vi "Controller Fast Command Loop.vi"(7 "Sync Objects":T1, 8 "error in (no error)":errorcluster, 11 "FOFB Configuration":T4={"FOFB Parameters"={"Network"={"FOFB Controller IP"="", "LNLS Control Network IP"="", "LNLS Control Network Power Supplies TCP Port"=0, "LNLS Control Network FOFB Configuration TCP Port"=0, "LNLS Control Network BPMs TCP Port"=0, "Data Server TCP Port"=0, "Monitoring Data TCP Port"=0, "Configuration GUI TCP Port"=0, "Storage Data TCP Port"=0, "Fast Command TCP Port"=0, "TCP Listening Timeout"=0, "Request Setpoints Rate"=0}, "Fast Acquisition"={"Acquisition Period"=0, "Data Buffer Size"=0, "Monitoring Period"=0}, "Response Matrix Measurement"={"Step Amplitude"=0.0, "Time Between Steps"=0, "Step Duration"=0, "Number of Averages"=0}, "Correction Algorithm"={"Correction Period"=0, "Reference Orbit Path"=path "", "Response Matrix Path"=path "", "Correction Matrix Path"=path "", "PID Horizontal Gain"=0.0, "PID Vertical Gain"=0.0, "PID Horizontal Integral Time"=0.0, "PID Vertical Integral Time"=0.0, "PID Horizontal Derivative Time"=0.0, "PID Vertical Derivative Time"=0.0, "Beam Current FOFB Threshold"=0.0, "Decouple H-V"=FALSE, "Use Additional BPM LPF"=FALSE, "BPM LPF Cutoff"=0.0}, "Acquisition Network"=[], "Actuation Network"=[]}, "Number of Acquisition Chassis"=0, "Number of Actuation Chassis"=0, "Number of BPM Readings"=0, "BPM Reading Names"=[], "Selected BPM Readings"=[0, 1, 2, 3, 4, 5, 6, 7, 8, 9, 10, 11, 12, 13, 14, 15, 16, 17, 18, 19, 20, 21, 22, 23, 24, 25, 26, 27, 28, 29, 30, 31, 32, 33, 34, 35, 36, 37, 38, 39, 40, 41, 42, 43, 44, 45, 46, 47, 48, 49], "Number of Correctors"=0, "Corrector Names"=[], "Selected Correctors"=[0, 1, 2, 3, 4, 5, 6, 7, 8, 9, 10, 11, 12, 13, 14, 15, 16, 17, 18, 19, 20, 21, 22, 23, 24, 25, 26, 27, 28, 29, 30, 31, 32, 33, 34, 35, 36, 37, 38, 39, 40, 41, 42, 43, 44, 45, 46, 47, 48, 49], "Reference Orbit"=[], "Response Matrix"=[], "Correction Matrix"=[], "Acquisition Chassis Names"=[], "Actuation Chassis Names"=[], "Acquisition Variables"=[], "Actuation Variables"=[], "PS Matrix Mapping"=[], "Inverse PS Matrix Mapping"=[], "BPM Matrix Mapping"=[], "Inverse BPM Matrix Mapping"=[], "Response Matrix Beam Energy (MeV)"=0.0, "PID Parameters"=[], "BPM Planes"=[], "Corrector Planes"=[], "RMM Step Factor"=[]}) -> (0 "error out":errorcluster)   [LabVIEW 2011, in "Controller VIs.lvlib"]
uses:
  Controller VIs.lvlib
  Types Definitions/Type FOFB Configuration.ctl
  Types Definitions/Type FOFB Parameters.ctl
  Types Definitions/Type Network Configuration.ctl
  Types Definitions/Type FA Configuration.ctl
  Types Definitions/Type Response Matrix Measurement Configuration.ctl
  Types Definitions/Type Correction Algorithm Configuration.ctl
  Types Definitions/Type Acquisition Network Configuration.ctl
  Types Definitions/Type Actuation Network Configuration.ctl
  Types Definitions/Type PID Parameters.ctl
  Types Definitions/Type Synchronization Objects.ctl
  Types Definitions/Type Blocking Synchronization Objects.ctl
  Types Definitions/Type Monitoring Data.ctl
  Types Definitions/Type Operation Mode State.ctl
  Types Definitions/Type Diagnostics Data.ctl
  Types Definitions/Type CPU Loads Array.ctl
  Types Definitions/Type CPU Loads.ctl
  Types Definitions/Type Non-blocking Synchronization Objects.ctl
  Types Definitions/Type FOFB Variables.ctl
  Types Definitions/Type Actuation State.ctl
  Types Definitions/Type TCP State.ctl
  <vilib>/Platform/TimedLoop/XDataNode/timing_clust.ctl
  <vilib>/Platform/TimedLoop/XDataNode/nitl_modes.ctl
  <vilib>/Platform/TimedLoop/XDataNode/wakeup.ctl
  <vilib>/Platform/TimedLoop/XDataNode/XDataNode.xnode
  Type Definitions.lvlib
  Misc VIs.lvlib
  <vilib>/Platform/TimedLoop/XDataNode/XDNodeRunTimeDep.lvlib
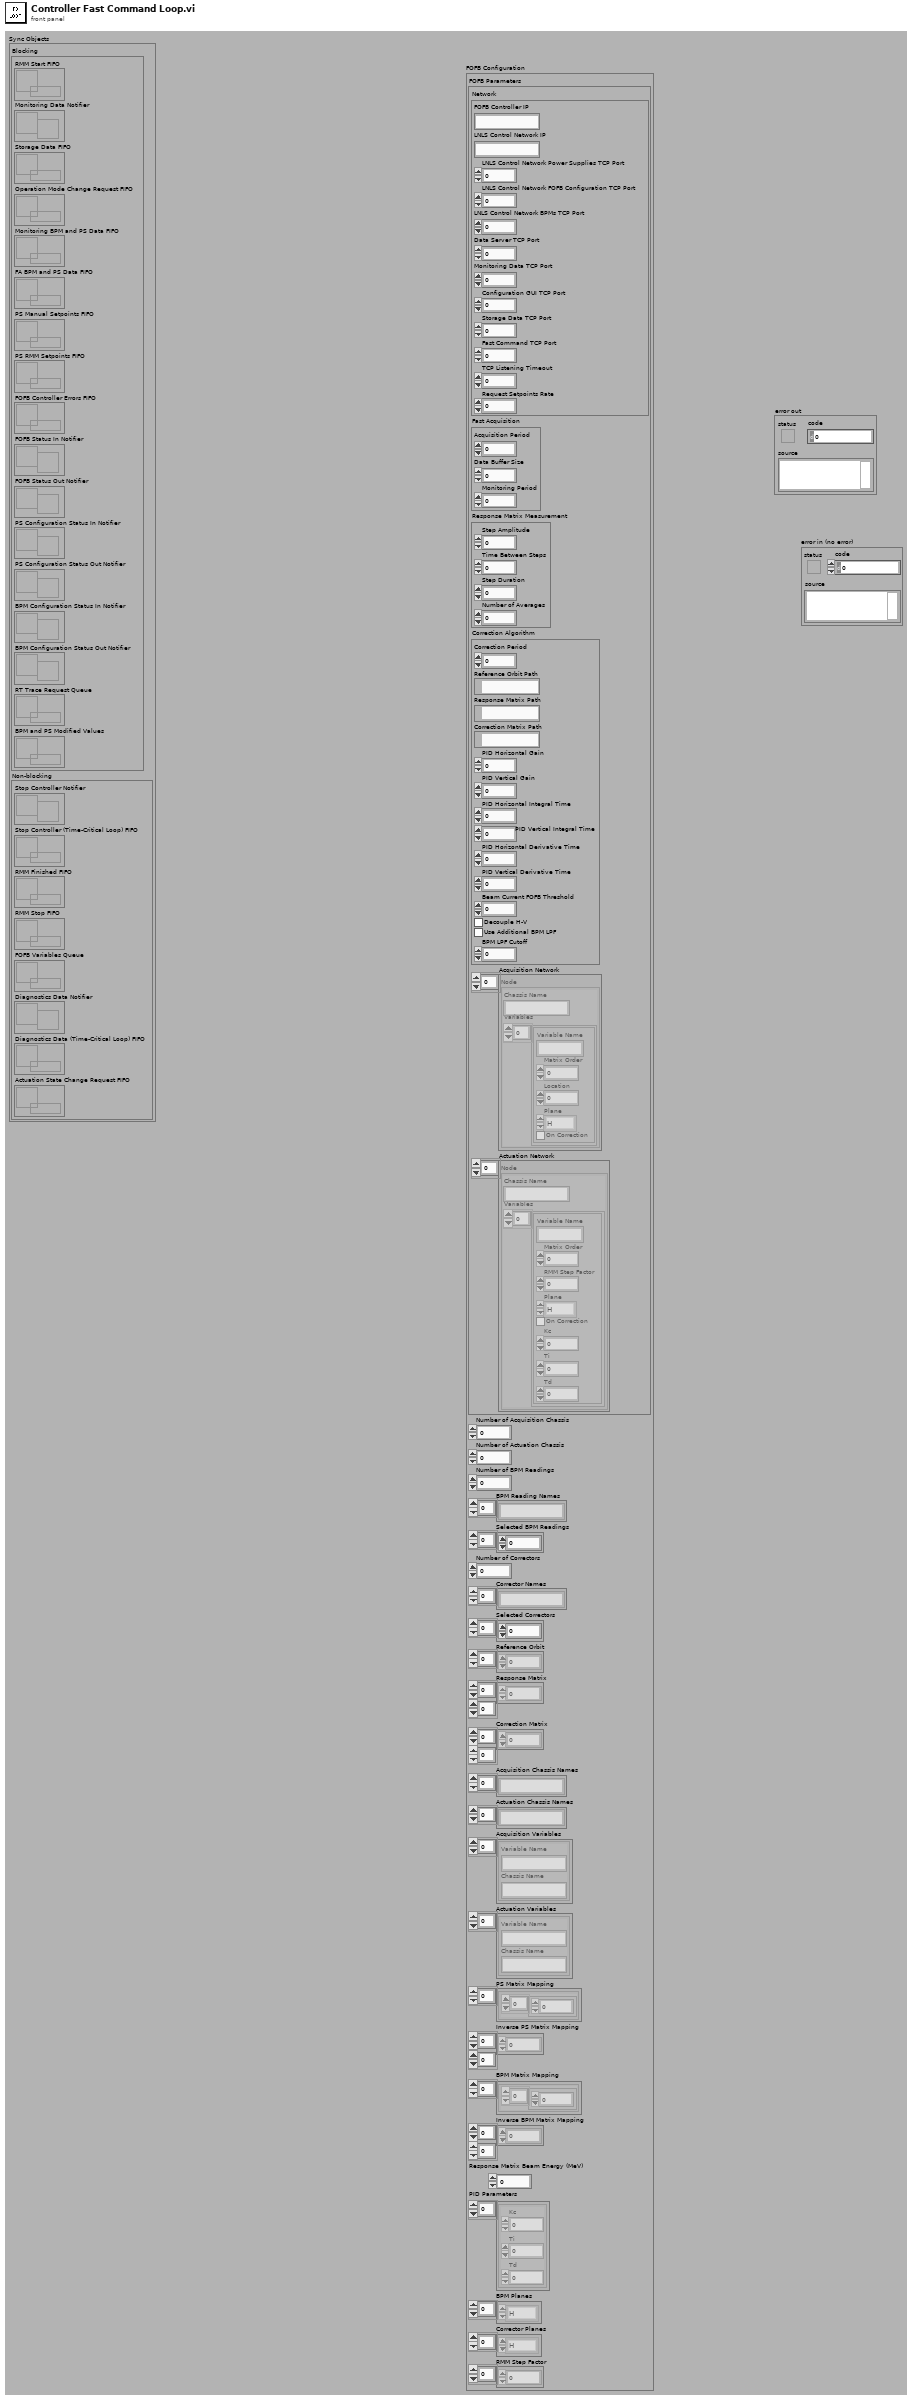
[diagram p1: front panel]
types:
  T1 = typedef "Type Definitions.lvlib/Type Synchronization Objects.ctl" = cluster{"Blocking":T2, "Non-blocking":T3}
  T2 = typedef "Type Definitions.lvlib/Type Blocking Synchronization Objects.ctl" = cluster{"RMM Start FIFO":refnum<k33>, "Monitoring Data Notifier":refnum<notifier>, "Storage Data FIFO":refnum<queue>, "Operation Mode Change Request FIFO":refnum<k33>, "Monitoring BPM and PS Data FIFO":refnum<k33>, "FA BPM and PS Data FIFO":refnum<k33>, "PS Manual Setpoints FIFO":refnum<k33>, "PS RMM Setpoints FIFO":refnum<k33>, "FOFB Controller Errors FIFO ":refnum<k33>, "FOFB Status In Notifier":refnum<notifier>, "FOFB Status Out Notifier":refnum<notifier>, "PS Configuration Status In Notifier":refnum<notifier>, "PS Configuration Status Out Notifier":refnum<notifier>, "BPM Configuration Status In Notifier":refnum<notifier>, "BPM Configuration Status Out Notifier":refnum<notifier>, "RT Trace Request Queue":refnum<queue>, "BPM and PS Modified Values":refnum<k33>}
  T3 = typedef "Type Definitions.lvlib/Type Non-blocking Synchronization Objects.ctl" = cluster{"Stop Controller Notifier":refnum<notifier>, "Stop Controller (Time-Critical Loop) FIFO":refnum<k33>, "RMM Finished FIFO":refnum<k33>, "RMM Stop FIFO":refnum<k33>, "FOFB Variables Queue":refnum<queue>, "Diagnostics Data Notifier":refnum<notifier>, "Diagnostics Data (Time-Critical Loop) FIFO":refnum<k33>, "Actuation State Change Request FIFO":refnum<k33>}
  T4 = typedef "Type Definitions.lvlib/Type FOFB Configuration.ctl" = cluster{"FOFB Parameters":T5, "Number of Acquisition Chassis":i32, "Number of Actuation Chassis":i32, "Number of BPM Readings":i32, "BPM Reading Names":string[], "Selected BPM Readings":u32[], "Number of Correctors":i32, "Corrector Names":string[], "Selected Correctors":u32[], "Reference Orbit":dbl[], "Response Matrix":dbl[][], "Correction Matrix":dbl[][], "Acquisition Chassis Names":string[], "Actuation Chassis Names":string[], "Acquisition Variables":cluster{"Variable Name":string, "Chassis Name":string}[], "Actuation Variables":cluster{"Variable Name":string, "Chassis Name":string}[], "PS Matrix Mapping":cluster{u32[]}[], "Inverse PS Matrix Mapping":u32[][], "BPM Matrix Mapping":cluster{u32[]}[], "Inverse BPM Matrix Mapping":u32[][], "Response Matrix Beam Energy (MeV)":dbl, "PID Parameters":T12[], "BPM Planes":enum8{"H", "V"}[], "Corrector Planes":enum8{"H", "V"}[], "RMM Step Factor":dbl[]}
  T5 = typedef "Type Definitions.lvlib/Type FOFB Parameters.ctl" = cluster{"Network":T6, "Fast Acquisition":T7, "Response Matrix Measurement":T8, "Correction Algorithm":T9, "Acquisition Network":T10, "Actuation Network":T11}
  T6 = typedef "Type Definitions.lvlib/Type Network Configuration.ctl" = cluster{"FOFB Controller IP":string, "LNLS Control Network IP":string, "LNLS Control Network Power Supplies TCP Port":u16, "LNLS Control Network FOFB Configuration TCP Port":u16, "LNLS Control Network BPMs TCP Port":u16, "Data Server TCP Port":u16, "Monitoring Data TCP Port":u16, "Configuration GUI TCP Port":u16, "Storage Data TCP Port":u16, "Fast Command TCP Port":u16, "TCP Listening Timeout":i32, "Request Setpoints Rate":u16}
  T7 = typedef "Type Definitions.lvlib/Type FA Configuration.ctl" = cluster{"Acquisition Period":u32, "Data Buffer Size":u32, "Monitoring Period":u32}
  T8 = typedef "Type Definitions.lvlib/Type Response Matrix Measurement Configuration.ctl" = cluster{"Step Amplitude":dbl, "Time Between Steps":u32, "Step Duration":u32, "Number of Averages":u32}
  T9 = typedef "Type Definitions.lvlib/Type Correction Algorithm Configuration.ctl" = cluster{"Correction Period":u32, "Reference Orbit Path":path, "Response Matrix Path":path, "Correction Matrix Path":path, "PID Horizontal Gain":dbl, "PID Vertical Gain":dbl, "PID Horizontal Integral Time":dbl, "PID Vertical Integral Time":dbl, "PID Horizontal Derivative Time":dbl, "PID Vertical Derivative Time":dbl, "Beam Current FOFB Threshold":dbl, "Decouple H-V":bool, "Use Additional BPM LPF":bool, "BPM LPF Cutoff":dbl}
  T10 = typedef "Type Definitions.lvlib/Type Acquisition Network Configuration.ctl" = cluster{"Chassis Name":string, "Variables":cluster{"Variable Name":string, "Matrix Order":u32, "Location":dbl, "Plane":enum8{"H", "V"}, "On Correction":bool}[]}[]
  T11 = typedef "Type Definitions.lvlib/Type Actuation Network Configuration.ctl" = cluster{"Chassis Name":string, "Variables":cluster{"Variable Name":string, "Matrix Order":u32, "RMM Step Factor":dbl, "Plane":enum8{"H", "V"}, "On Correction":bool, "Kc":dbl, "Ti":dbl, "Td":dbl}[]}[]
  T12 = typedef "Type Definitions.lvlib/Type PID Parameters.ctl" = cluster{"Kc":fxp<+/-,16,8>, "Ti":fxp<+/-,16,8>, "Td":fxp<+/-,16,8>}
  T13 = enum16{"big-endian, network order", "native, host order", "little-endian"}
  T14 = typedef "Type Definitions.lvlib/Type TCP State.ctl" = enum16{"Idle", "Wait Connection", "Read Data", "Process Data", "Write Data", "Close Connection"}
  T15 = typedef "XDNodeRunTimeDep.lvlib/timing_clust.ctl" = cluster{"Expected End [f-1]":u64, "Actual End [f-1]":u64, "Finished Late? [f-1]":bool, "Expected End [i-1]":u64, "Actual End [i-1]":u64, "Finished Late? [i-1]":bool, "Expected Start [i]":u64, "Actual Start [i]":u64, "Expected Start [f]":u64, "Actual Start [f]":u64, "Source Name":string, "Structure Name":string, "Period":i64, "Deadline":i64, "Offset":i64, "Start":i64, "Priority":i32, "Timeout":i32, "Mode":T16, "Wakeup Reason":T17, "Error":errorcluster, "Source Type":string, "Secondary Source Type":string, "Global End Time":u64, "Global Start Time":u64, "Frame Duration":u64, "Iteration Duration":u64, "Assigned CPU":i32, "I/O Scan Engine Mode":u32}
  T16 = typedef "XDNodeRunTimeDep.lvlib/nitl_modes.ctl" = enum32{"No Change", "Process missed periods, maintain original phase", "Discard missed periods, maintain original phase", "Process missed periods, ignore original phase", "Discard missed periods, ignore original phase"}
  T17 = typedef "XDNodeRunTimeDep.lvlib/wakeup.ctl" = enum32{"Normal", "Aborted", "Asynchronous wakeup", "Timing source error", "Timed loop error", "Timeout"}
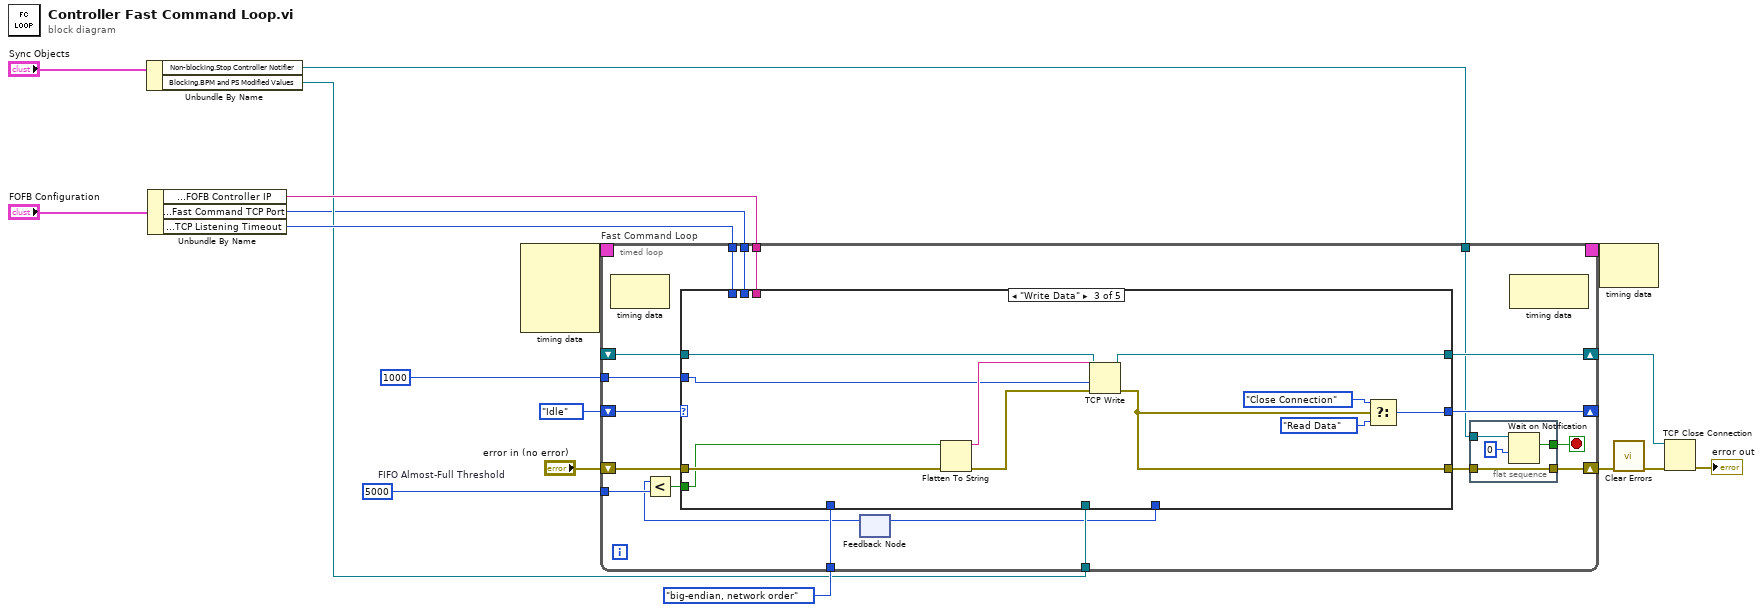
[diagram p0: block diagram]
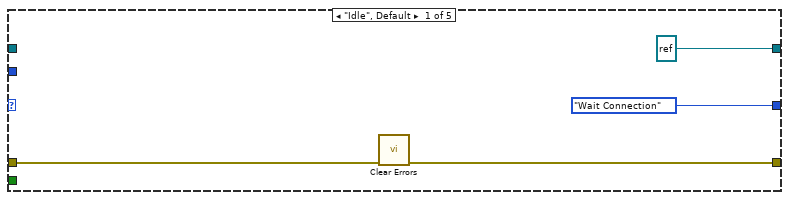
[diagram p2: hidden frame]
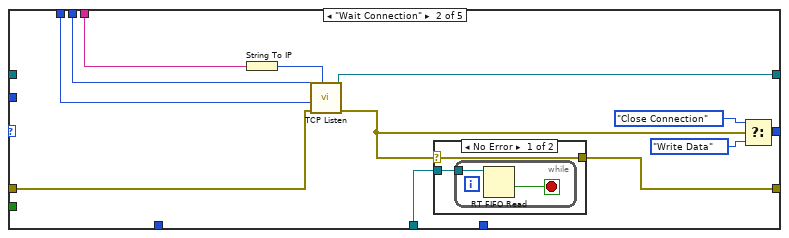
[diagram p3: hidden frame]
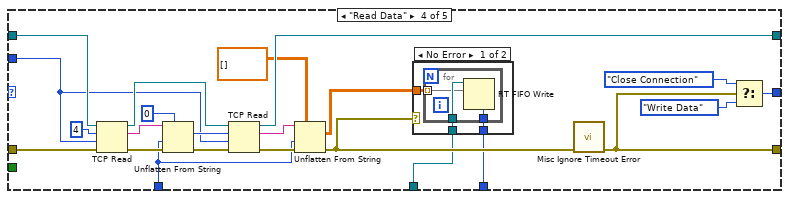
[diagram p5: hidden frame]
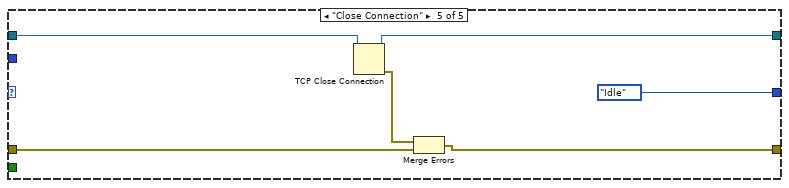
[diagram p7: hidden frame]
diagram:
  w12 = u32 5000  # FIFO Almost-Full Threshold
  n1 = Unbundle By Name("Sync Objects") -> ("Non-blocking.Stop Controller Notifier"=w5:refnum<notifier>, "Blocking.BPM and PS Modified Values"=w4:refnum<k33>)
  n2 = Unbundle By Name("FOFB Configuration") -> ("FOFB Parameters.Network.FOFB Controller IP"=w6:string, "FOFB Parameters.Network.Fast Command TCP Port"=w3:u16, "FOFB Parameters.Network.TCP Listening Timeout"=w7:i32)
  n3 = node-c288() -> (w17:T15)  [unwired: 4 in]
  n4 = timed-loop "Fast Command Loop" {
    tunnel: w6 -> [w37]
    tunnel: w3 -> [w36]
    tunnel: w7 -> [w35]
    shift-right: [w22] -> w11
    shift-left: "error in (no error)" -> [w30]
    shift-right: [w33] -> _
    shift-left: Type_TCP_State."Idle" ("f") -> [w34]
    shift-right: [w31] -> w13
    shift-left: _ -> [w32]
    timing: w17 -> [_]
    timing-out: [_] -> w16
    tunnel: T13."big-endian, network order" ("byte order (0:big-endian, network order)") -> [w29]
    tunnel: w4 -> [w28]
    tunnel: w12 -> [w27]
    tunnel: w5 -> [w20]
    tunnel: 1000 ("TCP Listening Timeout") -> [w19]
    stop <- w21 stop-if-true
    n5 = node-c288() -> ()  [unwired: 1 in, 1 out]
    n6 = feedback #1() -> (w25:u32)  [unwired: 1 in]
    n7 = Less?(x=w25, y=w27) -> (x < y?=w24:bool)
    n8 = case shown="\"Write Data\"" w34 {
      tunnel: [refnum<k5> refnum ("connection ID") w59 w75 w91 w110] -> w31
      tunnel: [Type_TCP_State."Wait Connection" ("f") w58 w74 w87 Type_TCP_State."Idle" ("f")] -> w33
      tunnel: [w44 w49 w72 w82 w105] -> w23
      tunnel: w30 -> [w45 w55 w71 w90 w106]
      tunnel: w32 -> [_ _ w68 w93 w108]
      tunnel: w37 -> [_ w52 _ _ _]
      tunnel: w36 -> [_ w54 _ _ _]
      tunnel: w35 -> [_ w48 _ _ _]
      tunnel: w29 -> [_ _ _ w77 _]
      tunnel: w24 -> [_ _ w67 _ _]
      tunnel: w28 -> [_ w51 _ w79 _]
      tunnel: [_ _ _ w78 _] -> w26
      tunnel: w19 -> [_ _ w65 w76 _]
      frame "Idle", Default {
        n9 = call <vilib>:"Clear Errors.vi"("error in (no error)"=w45) -> ("error out"=w44:errorcluster)  [unwired: 6 in]
      }
      frame "Wait Connection" {
        n10 = String To IP(1:w52) -> (0:w53:u32)
        n11 = call <vilib>:"TCP Listen.vi"("net address"=w53, "error in (no error)"=w55, "timeout ms (wait forever: -1)"=w48, "port"=w54) -> ("error out"=w50:errorcluster, "connection ID"=w59:refnum<k5>)  [unwired: 3 in, 3 out]
        n12 = case shown="No Error" w50 {
          selector: w50 -> [w60 w64]
          tunnel: w51 -> [w61 _]
          tunnel: [w60 w64] -> w49
          frame No Error {
            n13 = while {
              tunnel: w61 -> [w63]
              stop <- w62 stop-if-true
              n14 = RT FIFO Read(0:w63) -> (10:w62:bool)  [unwired: 3 in, 4 out]
            }
          }
          frame Error {
          }
        }
        n15 = Select(t=Type_TCP_State."Close Connection" ("f"), s=w50, f=Type_TCP_State."Write Data") -> (s? t:f=w58:T14)
      }
      frame "Write Data" {
        n16 = Flatten To String(anything=w67, error in (no error)=w71) -> (data string=w69:string, error out=w70:errorcluster)  [unwired: 2 in, 1 out]
        n17 = TCP Write(connection ID=w68, data in=w69, error in (no error)=w70, 9:w65) -> (connection ID out=w75:refnum<k5>, error out=w72:errorcluster)  [unwired: 1 out]
        n18 = Select(t=Type_TCP_State."Close Connection" ("f"), s=w72, f=Type_TCP_State."Read Data") -> (s? t:f=w74:T14)
      }
      frame "Read Data" {
        n19 = TCP Read(connection ID=w93, bytes to read=4, error in (no error)=w90, 9:w76) -> (connection ID out=w92:refnum<k5>, data out=w98:string, error out=w96:errorcluster)  [unwired: 1 in]
        n20 = Unflatten From String(type=0 ("length"), binary string=w98, byte order (0:big-endian, network order)=w77, error in (no error)=w96) -> (value=w83:i32, error out=w95:errorcluster)  [unwired: 1 in, 1 out]
        n21 = TCP Read(connection ID=w92, bytes to read=w83, error in (no error)=w95, 9:w76) -> (connection ID out=w91:refnum<k5>, data out=w81:string, error out=w94:errorcluster)  [unwired: 1 in]
        n22 = Unflatten From String(type=sgl[][] [], binary string=w81, byte order (0:big-endian, network order)=w77, error in (no error)=w94) -> (value=w85:sgl[][], error out=w80:errorcluster)  [unwired: 1 in, 1 out]
        n23 = case shown="No Error" w80 {
          tunnel: w85 -> [w101 _]
          tunnel: w79 -> [w100 _]
          tunnel: [w99 _] -> w78
          frame No Error {
            n24 = for {
              tunnel: w101 -> [w102] mode=indexing
              tunnel: w100 -> [w104]
              tunnel: [w103] -> w99
              n25 = RT FIFO Write(0:w104, 1:w102) -> (7:w103:u32)  [unwired: 3 in, 3 out]
            }
          }
          frame Error {
          }
        }
        n26 = call "Misc Ignore Timeout Error.vi"("error in (no error)"=w80) -> ("error out"=w82:errorcluster)  [unwired: 9 in, 1 out]
        n27 = Select(t=Type_TCP_State."Close Connection" ("f"), s=w82, f=Type_TCP_State."Write Data") -> (s? t:f=w87:T14)
      }
      frame "Close Connection" {
        n28 = TCP Close Connection(connection ID=w108) -> (connection ID out=w110:refnum<k5>, error out=w107:errorcluster)  [unwired: 2 in]
        n29 = Merge Errors(w107, w106) -> (w105:errorcluster)
      }
    }
    n30 = feedback-in #1(w26) -> ()
    n31 = flat-sequence {
      tunnel: [w40] -> w21
      tunnel: w20 -> [w39]
      tunnel: [w38] -> w22
      tunnel: w23 -> [w38]
      frame #0 {
        n32 = Wait on Notification(notifier=w39, timeout in ms (-1)=0) -> (notification=w40:bool)  [unwired: 2 in, 3 out]
      }
    }
    n33 = node-c288() -> ()  [unwired: 1 in, 1 out]
  }
  n34 = node-c288(w16) -> ()  [unwired: 1 out]
  n35 = call <vilib>:"Clear Errors.vi"("error in (no error)"=w11) -> ("error out"=w10:errorcluster)  [unwired: 6 in]
  n36 = TCP Close Connection(connection ID=w13, error in (no error)=w10) -> (error out=→"error out":errorcluster)  [unwired: 1 in, 1 out]
